vi "GEA2 Message to HEUI_LEDs.vi"(0 "Ignore Brightness?":bool, 7 "Raw Data In":string) -> (8 "HEUI_LEDs":T1)   [LabVIEW 2016, in "TL27.lvlib"]
uses:
  Projects/TL27.lvlib
  controls/HEUI_LEDs.ctl
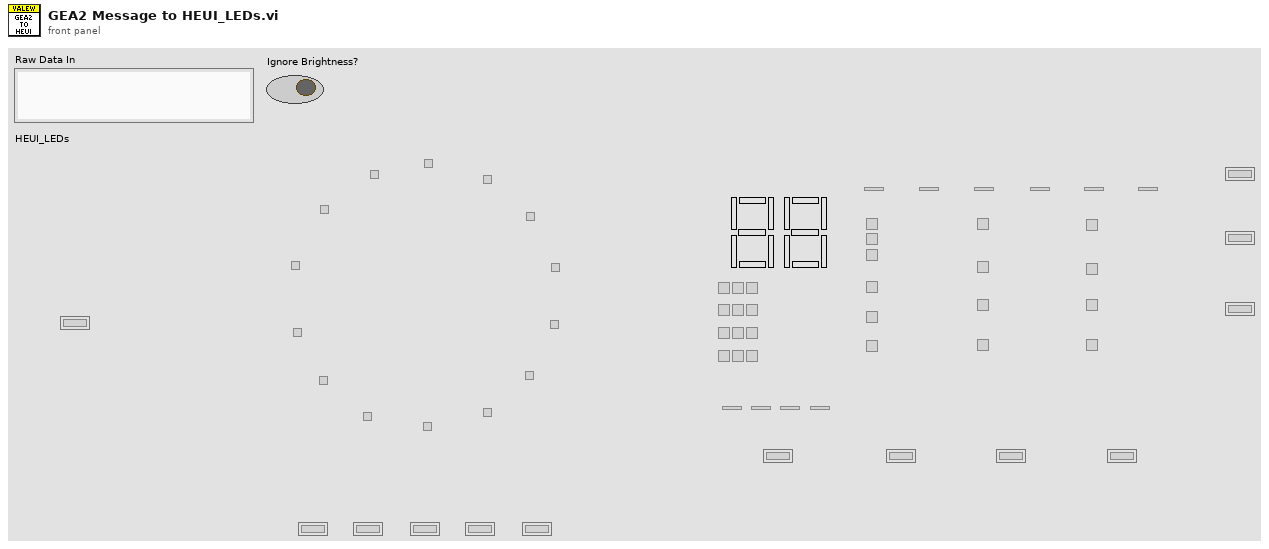
[diagram p1: front panel]
types:
  T1 = typedef "TL27.lvlib/HEUI_LEDs.ctl" = cluster{"Z101 - Start":bool, "Z103 - Colors":bool, "Z104 - Whites":bool, "Z105 - Towels":bool, "Z106 - Bulky Items":bool, "Z107 - Heavy Duty":bool, "Z108 - Jeans":bool, "Z109 - Basket Clean":bool, "Z110 - Drain and Spin":bool, "Z111 - Rinse and Spin":bool, "Z112 - Speed Wash":bool, "Z113 - Active Wear":bool, "Z114 - Hand Wash":bool, "Z115 - Delicates":bool, "Z116 - Easy Care":bool, "Z117 - Tomato":bool, "Z118 - Wine":bool, "Z119 - Blood":bool, "Z120 - Grass":bool, "Z121 - Dirt":bool, "Z122_MSB_A":bool, "Z123_MSB_B":bool, "Z124_MSB_G":bool, "Z125_MSB_C":bool, "Z126_MSB_D":bool, "Z127_MSB_E":bool, "Z128_MSB_F":bool, "Z129_LSB_A":bool, "Z130_LSB_B":bool, "Z131_LSB_G":bool, "Z132_LSB_C":bool, "Z133_LSB_D":bool, "Z134_LSB_E":bool, "Z135_LSB_F":bool, "Z136 - Pause":bool, "Z137 - Pause":bool, "Z138 - Lock Controls":bool, "Z139 - Lock Controls":bool, "Z140 - Lock Controls":bool, "Z141 - Lid Lock":bool, "Z142 - Lid Lock":bool, "Z143 - Lid Lock":bool, "Z144 - Good":bool, "Z145":bool, "Z146":bool, "Z147 - Better":bool, "Z148 - Delay":bool, "Z149 - Fill":bool, "Z150 - Soak":bool, "Z151 - Wash":bool, "Z152 - Rinse":bool, "Z153 - Spin":bool, "Z154 - Hot":bool, "Z155 - Warm":bool, "Z156 - Colors":bool, "Z157 - Cool":bool, "Z158 - Cold":bool, "Z159 - Tap Cold":bool, "Z160 - Extra Heavy":bool, "Z161 - Heavy":bool, "Z162 - Normal":bool, "Z163 - Light":bool, "Z164 - Max Spin":bool, "Z165 - More Spin":bool, "Z166 - Normal Spin":bool, "Z167 - No Spin":bool, "Z168 - Extra Rinse":bool, "Z170 - Deep Rinse":bool, "Z171 - Auto Soak":bool, "Z172 - Warm Rinse":bool, "Z173 - Deep Fill":bool, "Z174 - My Cycles":bool, "Z175 - Delay Wash":bool, "Z176 - Spin Stop":bool, "Z177 - Spin Stop":bool, "Z178 - Spin Stop":bool, "Z179 - Pause":bool, "Z109":bool, "Z110":bool, "Z123":bool, "Z124":bool, "Z140":bool, "Unused0":bool, "Unused1":bool, "Unused2":bool, "Unused3":bool, "Channel_Off":bool, "Channel_Cycle_Unmapped":bool}
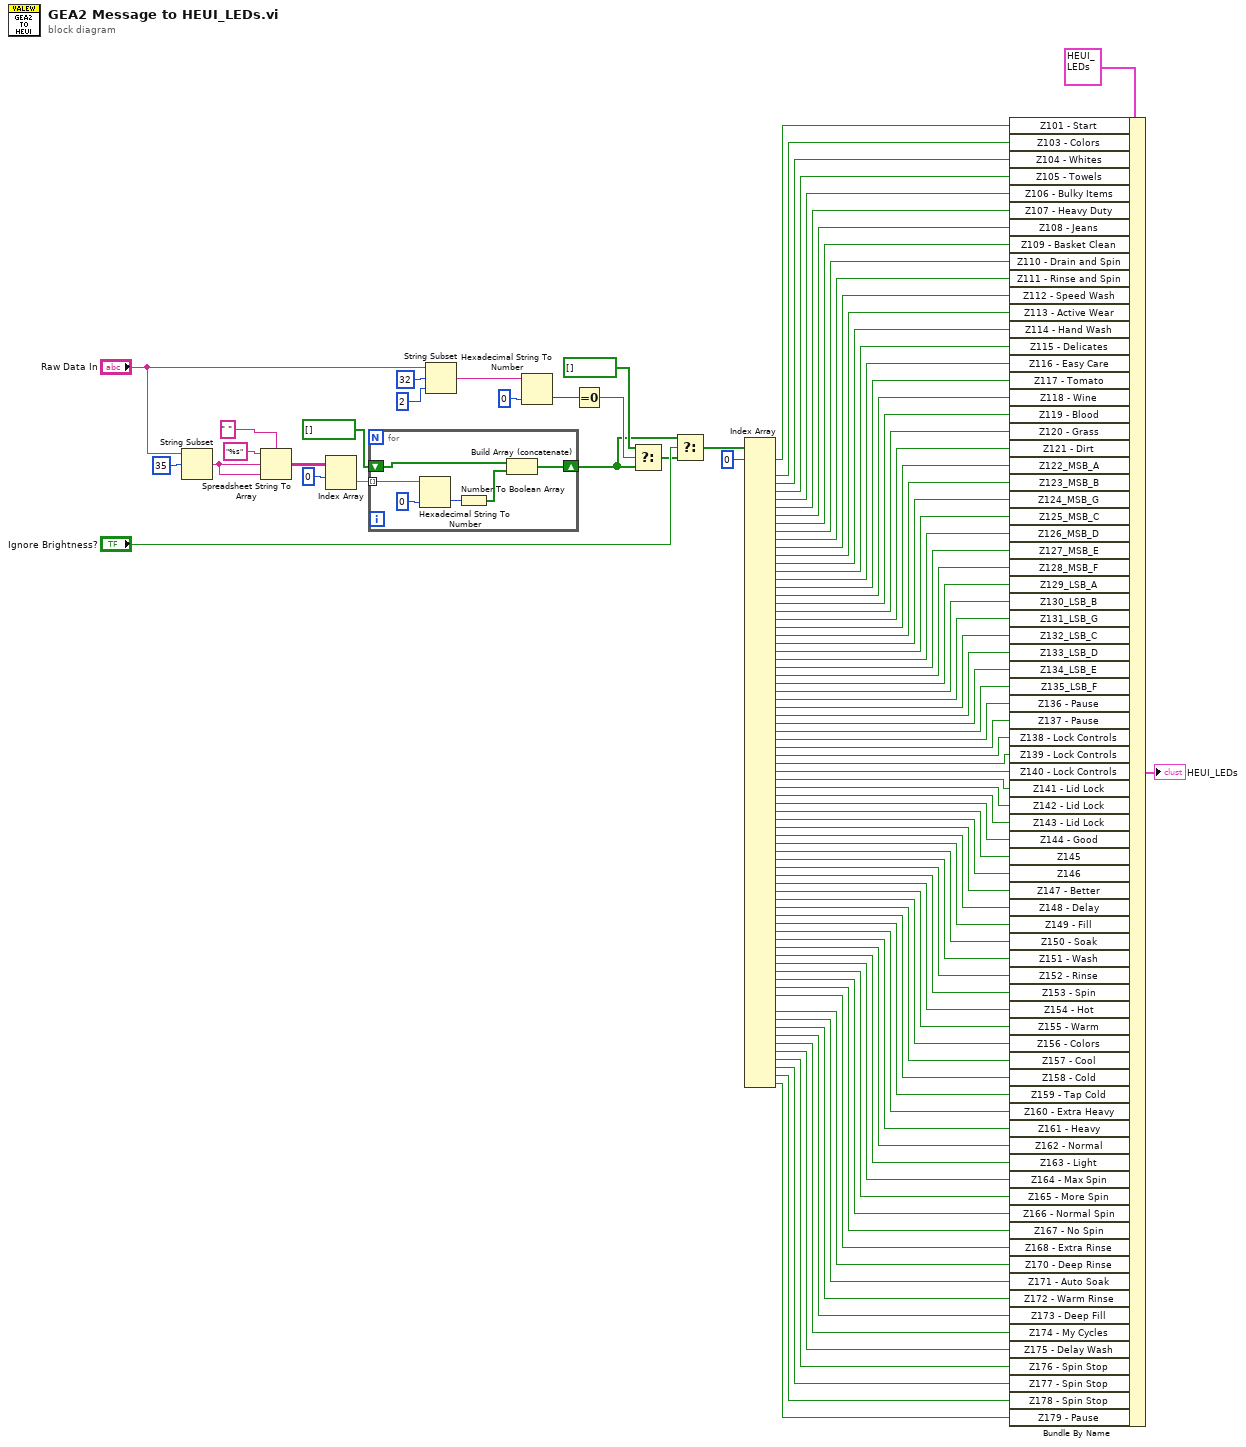
[diagram p0: block diagram]
diagram:
  n1 = String Subset(string="Raw Data In", offset (0)=35) -> (substring=w93:string)  [unwired: 1 in]
  n2 = Spreadsheet String To Array(delimiter (Tab)=" ", format string="%s", spreadsheet string=w93, array type (2D Dbl)=w93) -> (array=w97:string[][])
  n3 = Index Array(array=w97, index (row)=0) -> (element=w94:string[])  [unwired: 1 in]
  n4 = for {
    tunnel: w94 -> [w106] mode=indexing
    shift-right: [w102] -> w2
    shift-left: bool[] [] -> [w104]
    n5 = Hexadecimal String To Number(string=w106, default (0uL)=u8 0) -> (number=w105:u8)  [unwired: 1 in, 1 out]
    n6 = Number To Boolean Array(number=w105) -> (Boolean array=w103:bool[])
    n7 = Build Array (concatenate)(w104, w103) -> (w102:bool[])
  }
  n8 = String Subset(string="Raw Data In", offset (0)=32, length (rest)=2 ("length (rest)")) -> (substring=w90:string)
  n9 = Hexadecimal String To Number(string=w90, default (0uL)=u32 0 ("default (0 U32)")) -> (number=w88:u32)  [unwired: 1 in, 1 out]
  n10 = Equal To 0?(x=w88) -> (x = 0?=w87:bool)
  n11 = Select(t=bool[] [], s=w87, f=w2) -> (s? t:f=w1:bool[])
  n12 = Select(t=w2, s="Ignore Brightness?", f=w1) -> (s? t:f=w4:bool[])
  n13 = Index Array(array=w4, index #1=0 ("index")) -> (element #1=w85:bool, element #3=w83:bool, element #4=w82:bool, element #5=w81:bool, element #6=w80:bool, element #7=w79:bool, element #8=w78:bool, element #9=w77:bool, element #10=w76:bool, element #11=w75:bool, element #12=w74:bool, element #13=w73:bool, element #14=w72:bool, element #15=w71:bool, element #16=w70:bool, element #17=w69:bool, element #18=w68:bool, element #19=w66:bool, element #20=w65:bool, element #21=w64:bool, element #22=w63:bool, element #23=w62:bool, element #24=w61:bool, element #25=w60:bool, element #26=w59:bool, element #27=w58:bool, element #28=w57:bool, element #29=w56:bool, element #30=w55:bool, element #31=w54:bool, element #32=w53:bool, element #33=w52:bool, element #34=w51:bool, element #35=w50:bool, element #36=w49:bool, element #37=w48:bool, element #38=w47:bool, element #39=w46:bool, element #40=w45:bool, element #41=w44:bool, element #42=w43:bool, element #43=w42:bool, element #44=w41:bool, element #45=w40:bool, element #46=w39:bool, element #47=w38:bool, element #48=w37:bool, element #49=w36:bool, element #50=w35:bool, element #51=w34:bool, element #52=w33:bool, element #53=w32:bool, element #54=w31:bool, element #55=w30:bool, element #56=w29:bool, element #57=w28:bool, element #58=w27:bool, element #59=w26:bool, element #60=w25:bool, element #61=w24:bool, element #62=w23:bool, element #63=w22:bool, element #64=w21:bool, element #65=w20:bool, element #66=w19:bool, element #67=w18:bool, element #68=w7:bool, element #70=w8:bool, element #71=w9:bool, element #72=w10:bool, element #73=w11:bool, element #74=w12:bool, element #75=w13:bool, element #76=w14:bool, element #77=w15:bool, element #78=w16:bool, element #79=w17:bool)  [unwired: 78 in, 2 out]
  n14 = Bundle By Name(cluster=T1 {"Z101 - Start"=FALSE, "Z103 - Colors"=FALSE, "Z104 - Whites"=FALSE, "Z105 - Towels"=FALSE, "Z106 - Bulky Items"=FALSE, "Z107 - Heavy Duty"=FALSE, "Z108 - Jeans"=FALSE, "Z109 - Basket Clean"=FALSE, "Z110 - Drain and Spin"=FALSE, "Z111 - Rinse and Spin"=FALSE, "Z112 - Speed Wash"=FALSE, "Z113 - Active Wear"=FALSE, "Z114 - Hand Wash"=FALSE, "Z115 - Delicates"=FALSE, "Z116 - Easy Care"=FALSE, "Z117 - Tomato"=FALSE, "Z118 - Wine"=FALSE, "Z119 - Blood"=FALSE, "Z120 - Grass"=FALSE, "Z121 - Dirt"=FALSE, "Z122_MSB_A"=FALSE, "Z123_MSB_B"=FALSE, "Z124_MSB_G"=FALSE, "Z125_MSB_C"=FALSE, "Z126_MSB_D"=FALSE, "Z127_MSB_E"=FALSE, "Z128_MSB_F"=FALSE, "Z129_LSB_A"=FALSE, "Z130_LSB_B"=FALSE, "Z131_LSB_G"=FALSE, "Z132_LSB_C"=FALSE, "Z133_LSB_D"=FALSE, "Z134_LSB_E"=FALSE, "Z135_LSB_F"=FALSE, "Z136 - Pause"=FALSE, "Z137 - Pause"=FALSE, "Z138 - Lock Controls"=FALSE, "Z139 - Lock Controls"=FALSE, "Z140 - Lock Controls"=FALSE, "Z141 - Lid Lock"=FALSE, "Z142 - Lid Lock"=FALSE, "Z143 - Lid Lock"=FALSE, "Z144 - Good"=FALSE, "Z145"=FALSE, "Z146"=FALSE, "Z147 - Better"=FALSE, "Z148 - Delay"=FALSE, "Z149 - Fill"=FALSE, "Z150 - Soak"=FALSE, "Z151 - Wash"=FALSE, "Z152 - Rinse"=FALSE, "Z153 - Spin"=FALSE, "Z154 - Hot"=FALSE, "Z155 - Warm"=FALSE, "Z156 - Colors"=FALSE, "Z157 - Cool"=FALSE, "Z158 - Cold"=FALSE, "Z159 - Tap Cold"=FALSE, "Z160 - Extra Heavy"=FALSE, "Z161 - Heavy"=FALSE, "Z162 - Normal"=FALSE, "Z163 - Light"=FALSE, "Z164 - Max Spin"=FALSE, "Z165 - More Spin"=FALSE, "Z166 - Normal Spin"=FALSE, "Z167 - No Spin"=FALSE, "Z168 - Extra Rinse"=FALSE, "Z170 - Deep Rinse"=FALSE, "Z171 - Auto Soak"=FALSE, "Z172 - Warm Rinse"=FALSE, "Z173 - Deep Fill"=FALSE, "Z174 - My Cycles"=FALSE, "Z175 - Delay Wash"=FALSE, "Z176 - Spin Stop"=FALSE, "Z177 - Spin Stop"=FALSE, "Z178 - Spin Stop"=FALSE, "Z179 - Pause"=FALSE, "Z109"=FALSE, "Z110"=FALSE, "Z123"=FALSE, "Z124"=FALSE, "Z140"=FALSE, "Unused0"=FALSE, "Unused1"=FALSE, "Unused2"=FALSE, "Unused3"=FALSE, "Channel_Off"=FALSE, "Channel_Cycle_Unmapped"=FALSE} ("HEUI_LEDs"), "Z101 - Start"=w85, "Z103 - Colors"=w83, "Z104 - Whites"=w82, "Z105 - Towels"=w81, "Z106 - Bulky Items"=w80, "Z107 - Heavy Duty"=w79, "Z108 - Jeans"=w78, "Z109 - Basket Clean"=w77, "Z110 - Drain and Spin"=w76, "Z111 - Rinse and Spin"=w75, "Z112 - Speed Wash"=w74, "Z113 - Active Wear"=w73, "Z114 - Hand Wash"=w72, "Z115 - Delicates"=w71, "Z116 - Easy Care"=w70, "Z117 - Tomato"=w69, "Z118 - Wine"=w68, "Z119 - Blood"=w66, "Z120 - Grass"=w65, "Z121 - Dirt"=w64, "Z122_MSB_A"=w63, "Z123_MSB_B"=w62, "Z124_MSB_G"=w61, "Z125_MSB_C"=w60, "Z126_MSB_D"=w59, "Z127_MSB_E"=w58, "Z128_MSB_F"=w57, "Z129_LSB_A"=w56, "Z130_LSB_B"=w55, "Z131_LSB_G"=w54, "Z132_LSB_C"=w53, "Z133_LSB_D"=w52, "Z134_LSB_E"=w51, "Z135_LSB_F"=w50, "Z136 - Pause"=w49, "Z137 - Pause"=w48, "Z138 - Lock Controls"=w47, "Z139 - Lock Controls"=w46, "Z140 - Lock Controls"=w45, "Z141 - Lid Lock"=w44, "Z142 - Lid Lock"=w43, "Z143 - Lid Lock"=w42, "Z144 - Good"=w41, "Z145"=w40, "Z146"=w39, "Z147 - Better"=w38, "Z148 - Delay"=w37, "Z149 - Fill"=w36, "Z150 - Soak"=w35, "Z151 - Wash"=w34, "Z152 - Rinse"=w33, "Z153 - Spin"=w32, "Z154 - Hot"=w31, "Z155 - Warm"=w30, "Z156 - Colors"=w29, "Z157 - Cool"=w28, "Z158 - Cold"=w27, "Z159 - Tap Cold"=w26, "Z160 - Extra Heavy"=w25, "Z161 - Heavy"=w24, "Z162 - Normal"=w23, "Z163 - Light"=w22, "Z164 - Max Spin"=w21, "Z165 - More Spin"=w20, "Z166 - Normal Spin"=w19, "Z167 - No Spin"=w18, "Z168 - Extra Rinse"=w7, "Z170 - Deep Rinse"=w8, "Z171 - Auto Soak"=w9, "Z172 - Warm Rinse"=w10, "Z173 - Deep Fill"=w11, "Z174 - My Cycles"=w12, "Z175 - Delay Wash"=w13, "Z176 - Spin Stop"=w14, "Z177 - Spin Stop"=w15, "Z178 - Spin Stop"=w16, "Z179 - Pause"=w17) -> (→"HEUI_LEDs":T1)
